vi "DFT based implementation of  linear convolution.vi"() -> ()   [LabVIEW 2009]
uses:
  <vilib>/Analysis/2dsp.llb/Inverse Complex FFT.vi
  <vilib>/Analysis/2dsp.llb/Real FFT.vi
  <vilib>/Analysis/2dsp.llb/1D Convolution (DBL).vi
  <vilib>/Analysis/NI_AALPro.lvlib
panel:
  out "Sequence x[n]":dbl[](graph)=[1.0, 6.123031769111886e-17, -1.0, -1.836909530733566e-16, 1.0, 3.061515884555943e-16, -1.0, -4.2861222383783204e-16, 1.0]
  out "y[n]= x[n]*h[n] (Linear Convolution)":dbl[](graph)=[1.0000000000000142, 2.000000000000014, 3.0, 6.0, 13.00000000000001, 26.000000000000007, 51.000000000000014, 102.0, 205.0, -102.0, -204.00000000000003, 103.99999999999996, 208.0, -95.99999999999994, -192.00000000000006, 127.99999999999989, 256.0]
  out "IFFT{X[k].H[k]}":dbl[](graph)=[-101.00000000000001, -202.00000000000003, 106.99999999999991, 214.0, -82.99999999999986, -166.00000000000003, 178.99999999999991, 358.0, 205.0]
  out "Sequence H[k]":cluster{dbl, "fundamental frequency":dbl, dbl[]}(graph)={0.0, "fundamental frequency"=1.0, [511.0, 140.45577997900753, -77.46806283596094, -146.0, -167.9877171430466, -167.9877171430466, -146.0, -77.46806283596094, 140.45577997900753]}
  out "Sequence h[n]":dbl[](graph)=[1.0, 2.0, 4.0, 8.0, 16.0, 32.0, 64.0, 128.0, 256.0]
  out "Sequence X[k]":cluster{dbl, "fundamental frequency":dbl, dbl[]}(graph)={0.0, "fundamental frequency"=1.0, [0.9999999999999997, 1.152703644666139, 3.3793852415718177, -0.5000000000000002, -0.03208888623795625, -0.03208888623795625, -0.5000000000000002, 3.3793852415718177, 1.152703644666139]}
  out "IFFT{X[k].H[k]} (Zero Padded x[n] & y[n])":dbl[](graph)=[0.9999999999998863, 1.9999999999998128, 3.0000000000004547, 6.000000000000093, 12.999999999999826, 25.999999999999652, 51.000000000000156, 102.00000000000027, 205.00000000000006, -102.00000000000027, -203.99999999999994, 104.0, 208.00000000000037, -96.00000000000009, -192.0000000000002, 127.9999999999997, 256.0000000000001]
  # "DFT - based implementation of the linear convolution of two finite-length sequences"
  # "Program developed by Indranil Sinharoy"
  # "Fig 1."
  # "Fig 5."
  # "Fig 6."
  # "Fig 4."
  # "Fig 3."
  # "Fig 2."
  # "Fig 7."
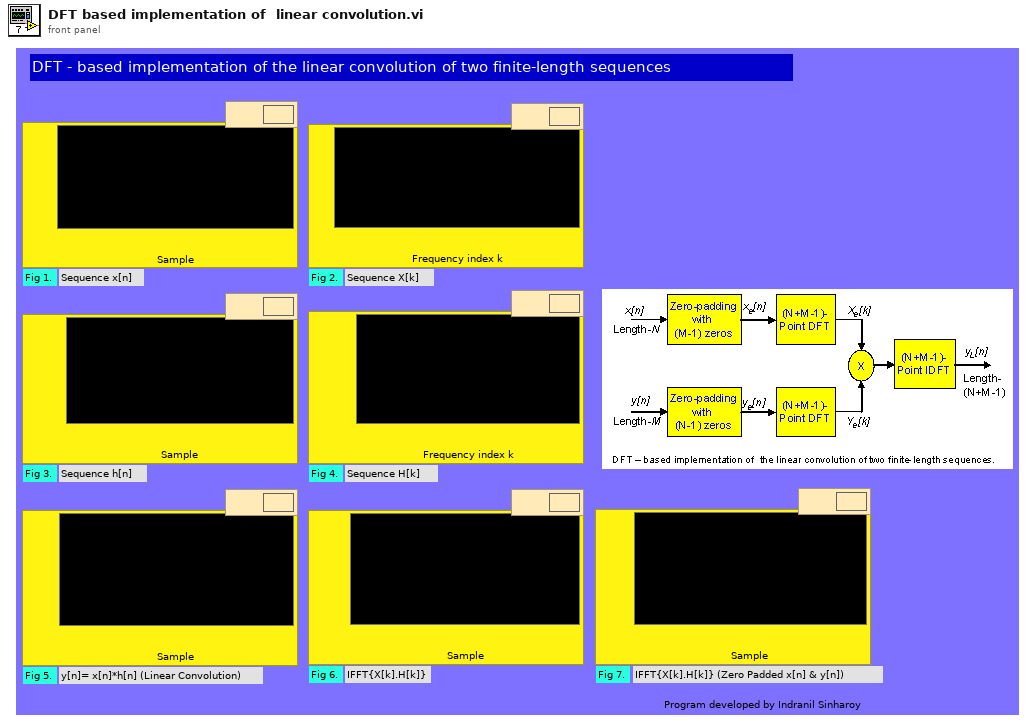
[diagram p1: front panel]
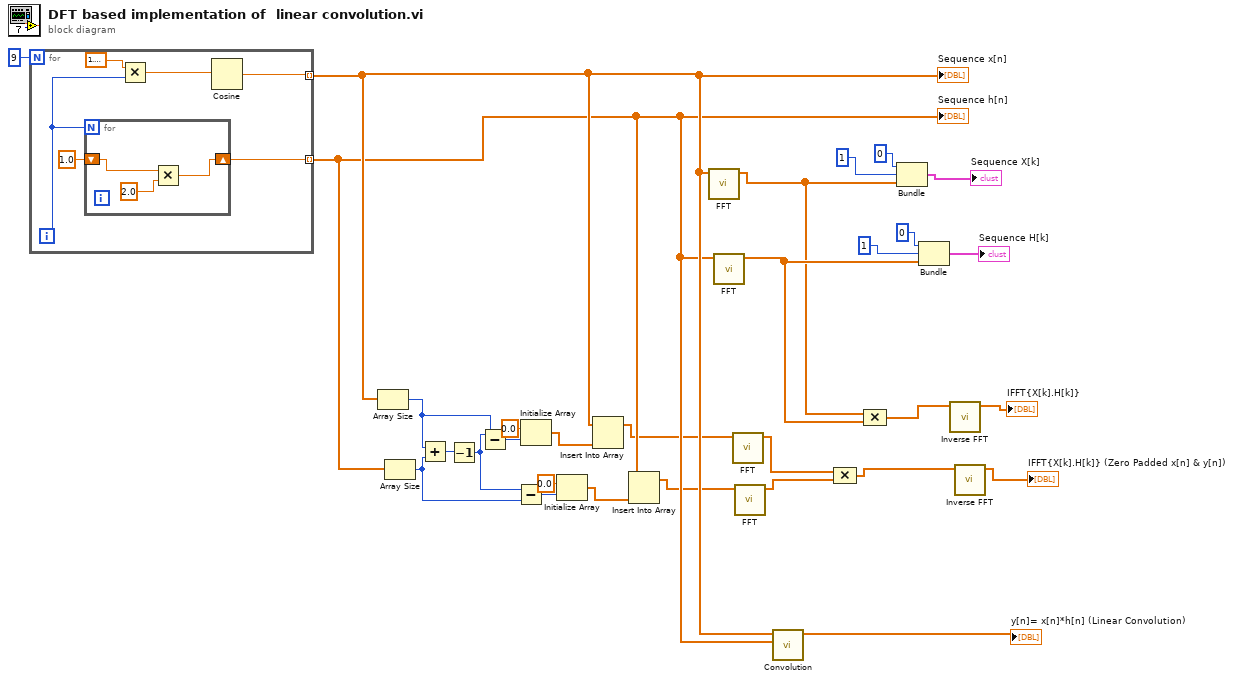
[diagram p0: block diagram]
diagram:
  n1 = for {
    N: 9 -> [_]
    tunnel: [w34] -> w14 mode=indexing
    tunnel: [w31] -> w10 mode=indexing
    i -> [w33]
    n2 = for {
      N: w33 -> [_]
      shift-right: [w38] -> w31
      shift-left: 1.0 -> [w37]
      n3 = Multiply(x=w37, y=2.0) -> (x*y=w38:dbl)
    }
    n4 = Multiply(x=1.5707963267948966, y=w33) -> (x*y=w35:dbl)
    n5 = Cosine(x=w35) -> (cos(x)=w34:dbl)
  }
  "Sequence x[n]" <- w14
  "Sequence h[n]" <- w10
  n6 = Array Size(array=w14) -> (size(s)=w3:i32)
  n7 = Array Size(array=w10) -> (size(s)=w1:i32)
  n8 = Add(x=w3, y=w1) -> (x+y=w18:i32)
  n9 = Decrement(x=w18) -> (x-1=w2:i32)
  n10 = Subtract(x=w2, y=w3) -> (x-y=w17:i32)
  n11 = Subtract(x=w2, y=w1) -> (x-y=w11:i32)
  n12 = Initialize Array(0.0 ("element"), w17) -> (w15:dbl[])
  n13 = Initialize Array(0.0 ("element"), w11) -> (w13:dbl[])
  n14 = Insert Into Array(array=w14, new element=w15) -> (w4:dbl[])  [unwired: 1 in]
  n15 = Insert Into Array(array=w10, new element=w13) -> (w9:dbl[])  [unwired: 1 in]
  n16 = call-poly <vilib>:"FFT.vi"("X"=w14) -> ("FFT {X}"=w19:cdb[])  [unwired: 9 in, 1 out]
  n17 = call-poly <vilib>:"FFT.vi"("X"=w10) -> ("FFT {X}"=w20:cdb[])  [unwired: 9 in, 1 out]
  n18 = call-poly <vilib>:"FFT.vi"("X"=w4) -> ("FFT {X}"=w8:cdb[])  [unwired: 9 in, 1 out]
  n19 = call-poly <vilib>:"FFT.vi"("X"=w9) -> ("FFT {X}"=w7:cdb[])  [unwired: 9 in, 1 out]
  n20 = call-poly <vilib>:"Convolution.vi"("Y"=w10, "X"=w14) -> ("X * Y"=→"y[n]= x[n]*h[n] (Linear Convolution)":dbl[])  [unwired: 8 in, 1 out]
  n21 = Compound Arithmetic op=MULTIPLY(w8, w7) -> (w6:cdb[])
  n22 = Compound Arithmetic op=MULTIPLY(w19, w20) -> (w28:cdb[])
  n23 = Bundle(0, 1, "FFT {X}"=w19) -> (→"Sequence X[k]":cluster{i32, i32, "FFT {X}":cdb[]})  [unwired: 1 in]
  n24 = Bundle(0, 1, "FFT {X}"=w20) -> (→"Sequence H[k]":cluster{i32, i32, "FFT {X}":cdb[]})  [unwired: 1 in]
  n25 = call-poly <vilib>:"Inverse FFT.vi"("FFT {X}"=w28) -> ("X"=→"IFFT{X[k].H[k]}":cdb[])  [unwired: 9 in, 1 out]
  n26 = call-poly <vilib>:"Inverse FFT.vi"("FFT {X}"=w6) -> ("X"=→"IFFT{X[k].H[k]} (Zero Padded x[n] & y[n])":cdb[])  [unwired: 9 in, 1 out]
